vi "Save Picture.vi"(0 "Save Image":bool, 1 "WaveformChart in":refnum<vi>) -> ()   [LabVIEW 2020]
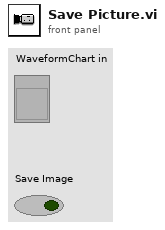
[diagram p1: front panel]
types:
  T1 = typedef "imagedata.ctl" = cluster{"image type":i32, "image depth":i32, "image":u8[], "mask":u8[], "colors":u32[], "Rectangle":cluster{"left":i16, "top":i16, "right":i16, "bottom":i16}}
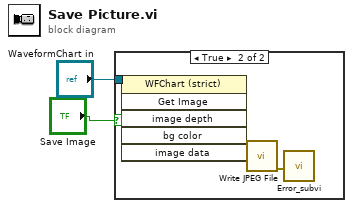
[diagram p0: block diagram]
diagram:
  n1 = case shown="True" "Save Image" {
    tunnel: "WaveformChart in" -> [_ w3]
    frame False {
    }
    frame True {
      n2 = invoke on="Invoke Node" class="WFChart (strict)" method="Get Image"(reference=w3) -> ("image data"=w5:T1)  [unwired: 5 in, 5 out]
      n3 = call <vilib>:"Write JPEG File.vi"("image data"=w5) -> ("error out"=w4:errorcluster)  [unwired: 9 in, 1 out]
      n4 = call "Error_subvi.vi"("error in (no error)"=w4) -> ()  [unwired: 3 out]
    }
  }
